vi "GENERATE SALE RECEIPT.vi"(11 "REFERENCES":T1) -> ()   [LabVIEW 2019]
uses:
  Controls/References Cluster.ctl
  <vilib>/userDefined/High Color/IMAQdx.ctl
  Controls/Custom Calendar/Custom Calendar.xctl
  <vilib>/addons/database/Auxilliary.llb/DB Tools Cursor Type.ctl
  <vilib>/Utility/NIReport.llb/Report Type.ctl
  <vilib>/addons/database/Connection.llb/DB Tools Open Connec (String).vi
  <vilib>/addons/database/Connection.llb/Conn Execute.vi
  <vilib>/addons/database/Recordset.llb/Rec Fetch Recordset Data (R).vi
  <vilib>/addons/database/Recordset.llb/Rec Destroy - Connection.vi
  <vilib>/Utility/NIReport.llb/Append Report Text (str wrap).vi
  <vilib>/Utility/NIReport.llb/Append Text Table to Report (wrap).vi
  <vilib>/addons/database/_DB Variant To Data/Database Variant To Data.xnode
  <vilib>/Utility/NIReport.llb/NI_report.lvclass
  <vilib>/Utility/NIReport.llb/NI_ReportGenerationCore.lvlib
  <vilib>/Utility/NIReport.llb/Word/NI_Word.lvclass
  <vilib>/addons/database/NI_Database_API.lvlib
types:
  T1 = typedef "References Cluster.ctl" = cluster{"MAIN PAGES":refnum<vi>, "ADD/EDIT ITEM REFERENCES":cluster{"Identifier":refnum<vi>, "BYU ICN #":refnum<vi>, "Item Description":refnum<vi>, "Comments":refnum<vi>, "Checked Out Date":refnum<vi>, "Due Date":refnum<vi>, "Check Out Location":refnum<vi>, "Reminder Count":refnum<vi>, "Most Recent Reminder Date":refnum<vi>, "BYU ID #":refnum<vi>, "Building/Room":refnum<vi>, "Location in Room":refnum<vi>, "Manual":refnum<vi>, "Manufacturer":refnum<vi>, "Model #":refnum<vi>, "Serial #":refnum<vi>, "Date Acquired":refnum<vi>, "ADD/EDIT ITEM LABEL":refnum<vi>, "ARCHIVE ITEM":refnum<vi>, "Archive Item Inputs":refnum<vi>, "Reminder Notes":refnum<vi>, "DUPLICATE ITEM":refnum<vi>}, "ADD/EDIT USER REFERENCES":cluster{"BYU ID # (##-###-####)":refnum<vi>, "First Name":refnum<vi>, "Last Name":refnum<vi>, "Phone Number (###-###-####)":refnum<vi>, "Email":refnum<vi>, "Department":refnum<vi>, "Graduation Status":refnum<vi>, "Anticipated Graduation Year":refnum<vi>, "Credit Score":refnum<vi>, "Date Added":refnum<vi>, "Graduation Clearance Date":refnum<vi>, "Picture File Name":refnum<vi>, "ADD/EDIT USER LABEL":refnum<vi>, "Department Map":refnum<vi>, "Status Map":refnum<vi>, "Anticipated Graduation Year Map":refnum<vi>, "User Agreement":refnum<vi>, "User Comments":refnum<vi>, "Camera":refnum<vi>}, "RETURN ITEM REFERENCES":cluster{"Item or Person:":refnum<vi>, "Search Return Results":refnum<vi>, "What are you searching for?":refnum<vi>}, "SEARCH DATABASE REFERENCES":cluster{"What to Search For:":refnum<vi>, "Where to Search":refnum<vi>, "Column to Search In":refnum<vi>, "Column to Sort By":refnum<vi>, "Search Database Results":refnum<vi>, "Inventory Column Selector":refnum<vi>, "User Column Selector":refnum<vi>, "Inventory Archive Column Selector":refnum<vi>, "User Archive Column Selector":refnum<vi>, "Sales Tracking Column Selector":refnum<vi>, "Checked In Archive Column Selector":refnum<vi>, "Restore User":refnum<vi>, "Date Range":refnum<vi>, "Dates Less Than":refnum<vi>, "Dates Greater Than":refnum<vi>, "Search Print Receipt":refnum<vi>, "Edit Sale Description":refnum<vi>}, "USER ITEMS REFERENCES":cluster{"USER'S INFORMATION":refnum<vi>, "User's Checked Out Items":refnum<vi>, "User Info Comments":refnum<vi>, "SEE USER INFO COMMENTS":refnum<vi>}, "EDIT ITEMS REFERENCES":cluster{"New Check Out Location":refnum<vi>, "Items to Edit":refnum<vi>, "Edit Items Due Date":refnum<vi>, "New Reminder Notes":refnum<vi>, "New Item Description":refnum<vi>}, "CHECK OUT ITEMS REFERENCES":cluster{"Enter Item:":refnum<vi>, "Check Out Items Due Date":refnum<vi>, "Check Out Location":refnum<vi>, "Items to be Checked Out":refnum<vi>, "Possible Items":refnum<vi>, "Altered Item Description":refnum<vi>}, "TRANSFER ITEMS REFERENCES":cluster{"Search Parameter":refnum<vi>, "What to Match":refnum<vi>, "Matching Individuals":refnum<vi>, "Items to be Transferred":refnum<vi>}, "SETTINGS REFERENCES":cluster{"PSC Database Settings":refnum<vi>, "PSC Sales Item Spreadsheet":refnum<vi>}, "PSC SALES REFERENCES":cluster{"BYU ID CARD #":refnum<vi>, "Sale Description":refnum<vi>, "Scan or Enter Item Name":refnum<vi>, "Items to be Sold":refnum<vi>, "Grand Total":refnum<vi>, "Item List":refnum<vi>}}
  T2 = typedef "NI_Database_API.lvlib/DB Tools Cursor Type.ctl" = enum16{"forward-only", "keyset", "dynamic", "static"}
  T3 = cluster{"position (excel)":cluster{"row":i32, "column":i32}, "name (excel)":string, "bookmark (word)":string}
  T4 = typedef "NI_ReportGenerationCore.lvlib/Report Type.ctl" = enum16{"HTML", "Word", "Excel"}
  T5 = enum16{"maximized", "minimized", "normal", "no change"}
  T6 = cluster{"BYU ID CARD #":refnum<vi>, "Sale Description":refnum<vi>, "Scan or Enter Item Name":refnum<vi>, "Items to be Sold":refnum<vi>, "Grand Total":refnum<vi>, "Item List":refnum<vi>}
  T7 = typedef "NI_Database_API.lvlib/Conn ObjectReference.ctl" = refnum<k1>
  T8 = typedef "NI_Database_API.lvlib/Rec ObjectReference.ctl" = refnum<k1>
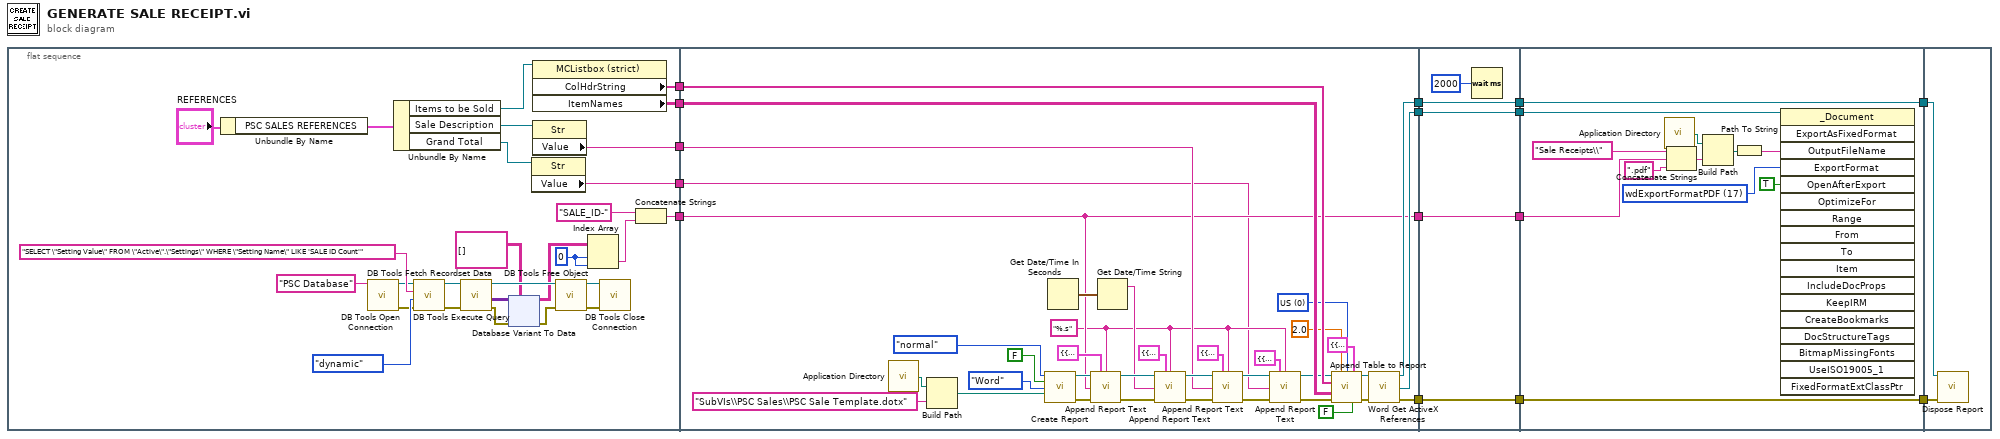
[diagram p0: block diagram]
diagram:
  n1 = flat-sequence {
    tunnel: [w26] -> w5
    tunnel: [w25] -> w4
    tunnel: [w24] -> w3
    tunnel: [w23] -> w2
    tunnel: [w16] -> w1
    tunnel: [w115] -> w15
    tunnel: [w111] -> w11
    tunnel: [w110] -> w8
    tunnel: [w98] -> w7
    tunnel: w5 -> [w100]
    tunnel: w4 -> [w101]
    tunnel: w3 -> [w99]
    tunnel: w2 -> [w98]
    tunnel: w1 -> [w91]
    tunnel: w15 -> [w129]
    tunnel: [w129] -> w14
    tunnel: [w127] -> w12
    tunnel: w11 -> [w127]
    tunnel: [w126] -> w9
    tunnel: w8 -> [w126]
    tunnel: w7 -> [w125]
    tunnel: [w125] -> w6
    tunnel: w14 -> [w130]
    tunnel: [w139] -> w13
    tunnel: w12 -> [w139]
    tunnel: [w138] -> w10
    tunnel: w9 -> [w138]
    tunnel: w6 -> [w135]
    tunnel: w13 -> [w143]
    tunnel: w10 -> [w142]
    frame #0 {
      w34 = 0 ("index")
      n2 = Unbundle By Name("REFERENCES") -> ("PSC SALES REFERENCES"=w30:T6)
      n3 = call-poly <vilib>:"DB Tools Open Connection.vi"("connection information"="PSC Database" ("string")) -> ("error out"=w21:errorcluster, "connection reference"=w22:T7)  [unwired: 7 in]
      n4 = Unbundle By Name(w30) -> ("Items to be Sold"=w27:refnum<vi>, "Sale Description"=w28:refnum<vi>, "Grand Total"=w17:refnum<vi>)
      n5 = call-poly <vilib>:"DB Tools Execute Query.vi"("error in (no error)"=w21, "cursor type"=DB_Tools_Cursor_Type."dynamic", "SQL query"="SELECT \"Setting Value\" FROM \"Active\".\"Settings\" WHERE \"Setting Name\" LIKE 'SALE ID Count'", "connection reference"=w22) -> ("error out"=w37:errorcluster, "recordset reference"=w36:T8)  [unwired: 4 in]
      n6 = call-poly <vilib>:"DB Tools Fetch Recordset Data.vi"("error in (no error)"=w37, "recordset reference"=w36) -> ("error out"=w39:errorcluster, "recordset data"=w38:variant[][], "recordset reference out"=w41:T8)  [unwired: 3 in]
      n7 = xnode "Database Variant To Data"("database variant"=w38, "error in (no error)"=w39, "type"=string[][] []) -> ("data"=w40:string[][], "error out"=w42:errorcluster)
      n8 = property class="Str"(reference=w17) -> ("Value"=w16:string)  [unwired: 1 in, 2 out]
      n9 = property class="MCListbox (strict)"(reference=w27) -> ("ColHdrString"=w25:string[], "ItemNames"=w26:string[][])  [unwired: 1 in, 2 out]
      n10 = property class="Str"(reference=w28) -> ("Value"=w24:string)  [unwired: 1 in, 2 out]
      n11 = call-poly <vilib>:"DB Tools Free Object.vi"("error in (no error)"=w42, "recordset reference"=w41) -> ("error out"=w19:errorcluster, "connection reference"=w18:T7)  [unwired: 8 in]
      n12 = Index Array(array=w40, index (row)=w34, index (col)=w34) -> (element=w43:string)
      n13 = call <vilib>:"DB Tools Close Connection.vi"("error in (no error)"=w19, "connection reference"=w18) -> ()  [unwired: 5 in, 1 out]
      n14 = Concatenate Strings("SALE_ID-" ("string"), w43) -> (w23:string)
    }
    frame #1 {
      w90 = u16 0 items=["US", "Metric", "Default"] ("measurement system")
      w92 = "%.s" ("format string (%.3f)")
      n15 = call <vilib>:"Application Directory.vi"() -> ("Application Directory"=w104:path)
      n16 = Build Path(base path=w104, name or relative path="SubVIs\\PSC Sales\\PSC Sale Template.dotx") -> (appended path=w102:path)
      n17 = call <vilib>:"Create Report.vi"("window state (normal)"=T5."normal", "display alerts? (F)"=FALSE, "report type"=Report_Type."Word", "template (empty)"=w102) -> ("report out"=w122:refnum<class "NI_report.lvclass">, "error out"=w121:errorcluster)  [unwired: 10 in]
      n18 = Get Date/Time In Seconds() -> (seconds since 1Jan1904=w106:timestamp)
      n19 = call-poly <vilib>:"Append Report Text.vi"("report in"=w122, "MS Office parameters"=T3 {"position (excel)"={"row"=0, "column"=0}, "name (excel)"="", "bookmark (word)"="Sale_ID"}, "format string (%.3f)"=w92, "text"=w98, "error in (no error)"=w121) -> ("report out"=w119:refnum<class "NI_report.lvclass">, "error out"=w118:errorcluster)  [unwired: 7 in, 2 out]
      n20 = Get Date/Time String(seconds (now)=w106) -> (date string=w105:string)  [unwired: 2 in, 1 out]
      n21 = call-poly <vilib>:"Append Report Text.vi"("report in"=w119, "MS Office parameters"=T3 {"position (excel)"={"row"=0, "column"=0}, "name (excel)"="", "bookmark (word)"="Sale_Date"}, "format string (%.3f)"=w92, "text"=w105, "error in (no error)"=w118) -> ("report out"=w114:refnum<class "NI_report.lvclass">, "error out"=w113:errorcluster)  [unwired: 7 in, 2 out]
      n22 = call-poly <vilib>:"Append Report Text.vi"("report in"=w114, "MS Office parameters"=T3 {"position (excel)"={"row"=0, "column"=0}, "name (excel)"="", "bookmark (word)"="Sale_Description"}, "format string (%.3f)"=w92, "text"=w99, "error in (no error)"=w113) -> ("report out"=w97:refnum<class "NI_report.lvclass">, "error out"=w96:errorcluster)  [unwired: 7 in, 2 out]
      n23 = call-poly <vilib>:"Append Report Text.vi"("report in"=w97, "MS Office parameters"=T3 {"position (excel)"={"row"=0, "column"=0}, "name (excel)"="", "bookmark (word)"="Sale_Grand_Total"}, "format string (%.3f)"=w92, "text"=w91, "error in (no error)"=w96) -> ("report out"=w95:refnum<class "NI_report.lvclass">, "error out"=w94:errorcluster)  [unwired: 7 in, 2 out]
      n24 = call-poly <vilib>:"Append Table to Report.vi"("report in"=w95, "column width (1)"=2.0, "measurement system"=w90, "MS Office parameters"=T3 {"position (excel)"={"row"=0, "column"=0}, "name (excel)"="", "bookmark (word)"="Sale_Items"}, "column headers"=w101, "text data"=w100, "error in (no error)"=w94, "show grid lines (YES)"=FALSE) -> ("report out"=w117:refnum<class "NI_report.lvclass">, "error out"=w116:errorcluster)  [unwired: 4 in, 2 out]
      n25 = call <vilib>:"Word Get ActiveX References.vi"("report in"=w117, "error in (no error)"=w116) -> ("report out"=w111:refnum<class "NI_report.lvclass">, "Word._Document"=w115:refnum<k7>, "error out"=w110:errorcluster)  [unwired: 7 in, 4 out]
    }
    frame #2 {
      n26 = Wait (ms)(milliseconds to wait=u32 2000) -> ()  [unwired: 1 out]
    }
    frame #3 {
      w141 = 17 items=["wdExportFormatPDF"=17, "wdExportFormatXPS"=18] ("ExportFormat")
      n27 = call <vilib>:"Application Directory.vi"() -> ("Application Directory"=w137:path)
      n28 = Concatenate Strings("Sale Receipts\\" ("name or relative path"), w135, ".pdf" ("name or relative path")) -> (w133:string)
      n29 = Build Path(base path=w137, name or relative path=w133) -> (appended path=w132:path)
      n30 = Path To String(path=w132) -> (string=w131:string)
      n31 = invoke class="_Document" method="ExportAsFixedFormat"(reference=w130, "OutputFileName"=w131, "ExportFormat"=w141, "OpenAfterExport"=TRUE) -> ()  [unwired: 14 in, 18 out]
    }
    frame #4 {
      n32 = call-dynamic "Dispose Report.vi"("report in"=w143, "error in (no error)"=w142) -> ()  [unwired: 13 in, 1 out]
    }
  }
